vi "N-565 Contol.vi"(0 "N-664 Notifier":refnum<notifier>, 5 "Stage Action":T1={"Action"=enum."Get Position", "Axis"=[], "Setpoint"=[], "Velocity"=0.5, "Cmd Recvd?"=FALSE, "Position"=[], "Status"=enum."Error", "Misc"=variant} {"Velocity" min=0.0 max=1.0 step=0.01}, 11 "VISA In":refnum<visa-resource-name>) -> (4 "N-664 Notifier (Dup)":refnum<notifier>)   [LabVIEW 2016]
uses:
  Stages Controls/Stage Notifier Element.ctl
  Stages Controls/Stage Actions.ctl
  Stages Controls/Stage Status.ctl
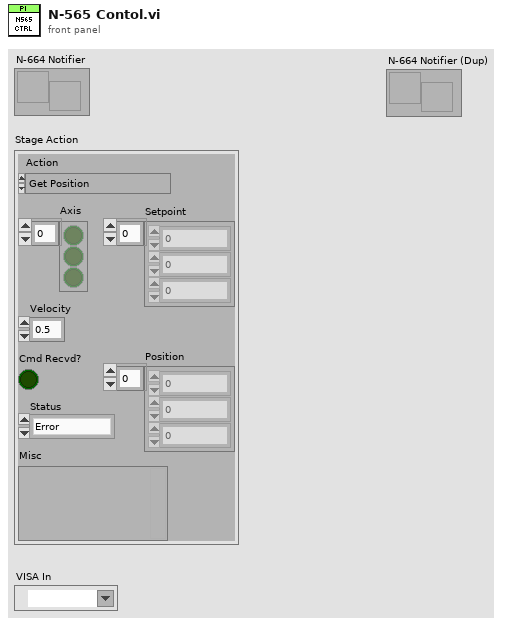
[diagram p1: front panel]
types:
  T1 = typedef "Stage Notifier Element.ctl" = cluster{"Action":T2, "Axis":bool[], "Setpoint":dbl[], "Velocity":dbl, "Cmd Recvd?":bool, "Position":dbl[], "Status":T3, "Misc":variant}
  T2 = typedef "Stage Actions.ctl" = enum16{"Get Position", "MVR", "MOVE", "HALT", "ONTARGET", "ERROR", "REFERENCE", "INIT", "VELOCITY", "STATUS", "EXIT", "HOME", "ZEROPOS", "NANOPOS", "ANALOG", "QUIT"}
  T3 = typedef "Stage Status.ctl" = enum16{"Error", "Abort", "Busy", "On Target"}
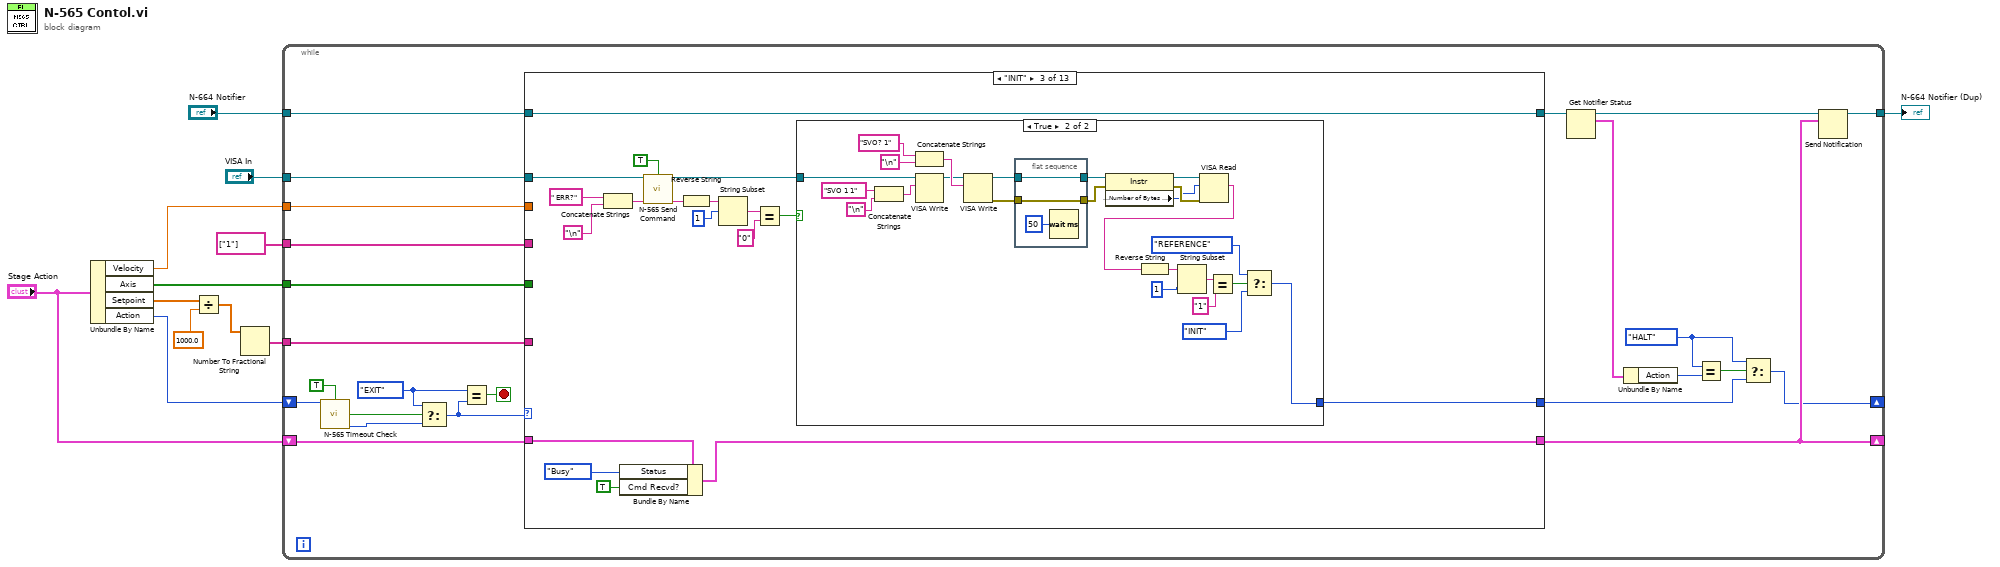
[diagram p0: block diagram]
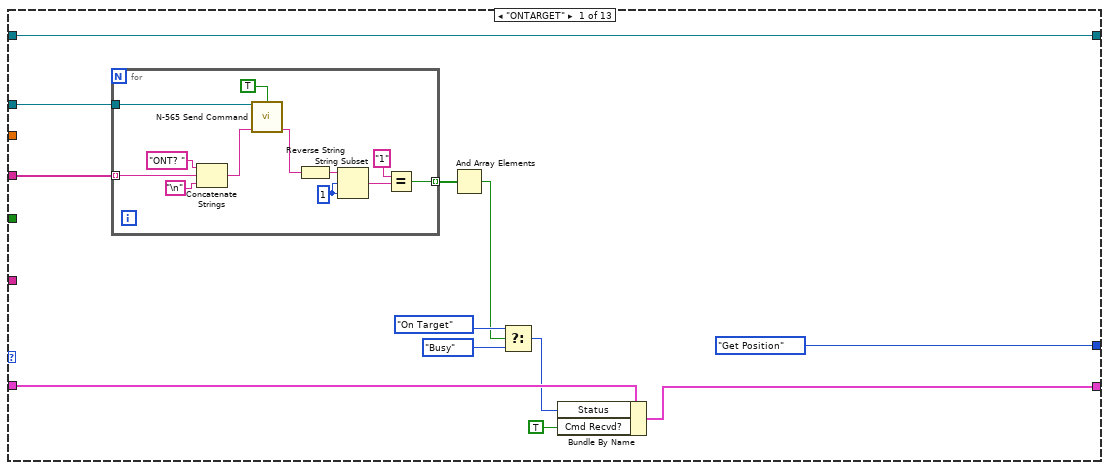
[diagram p2: hidden frame]
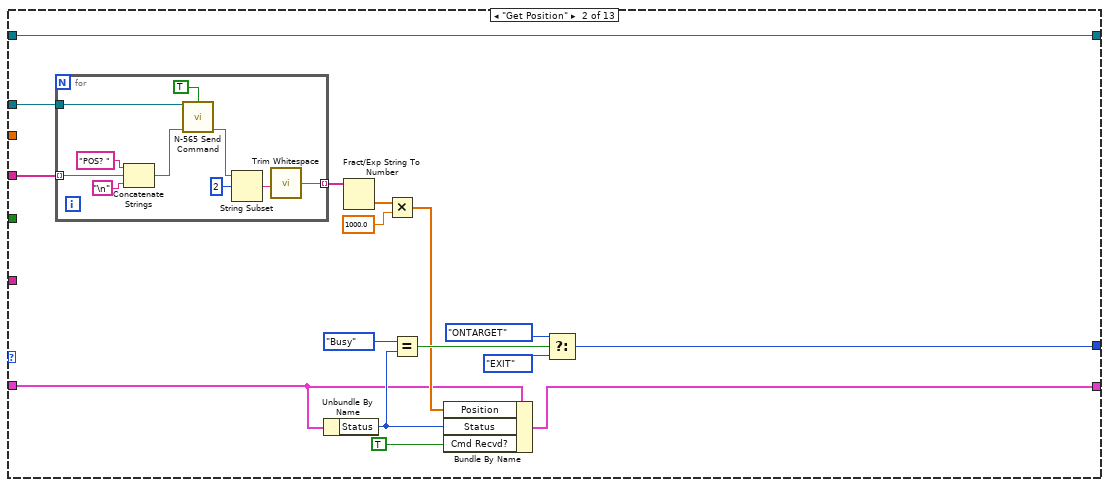
[diagram p3: hidden frame]
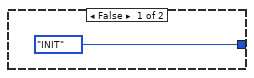
[diagram p4: hidden frame]
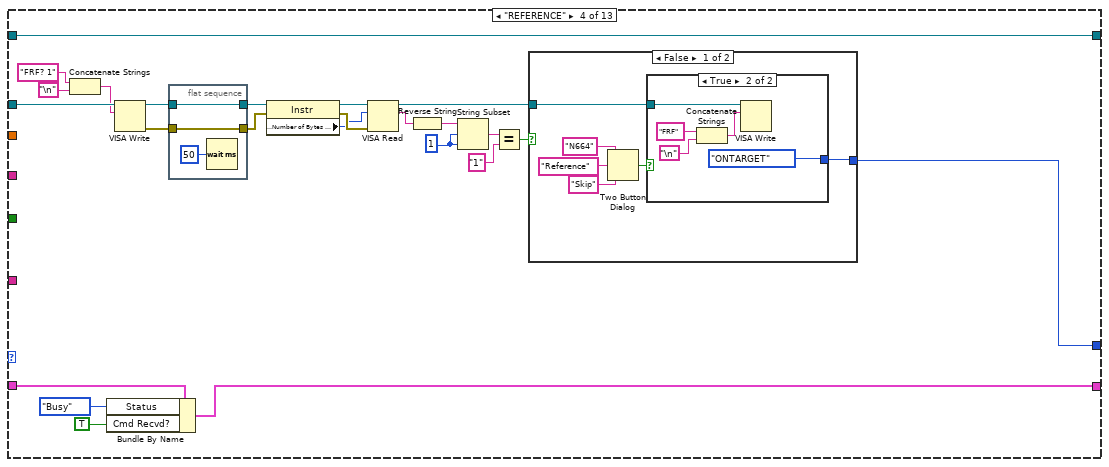
[diagram p5: hidden frame]
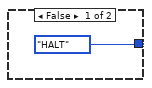
[diagram p6: hidden frame]
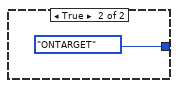
[diagram p7: hidden frame]
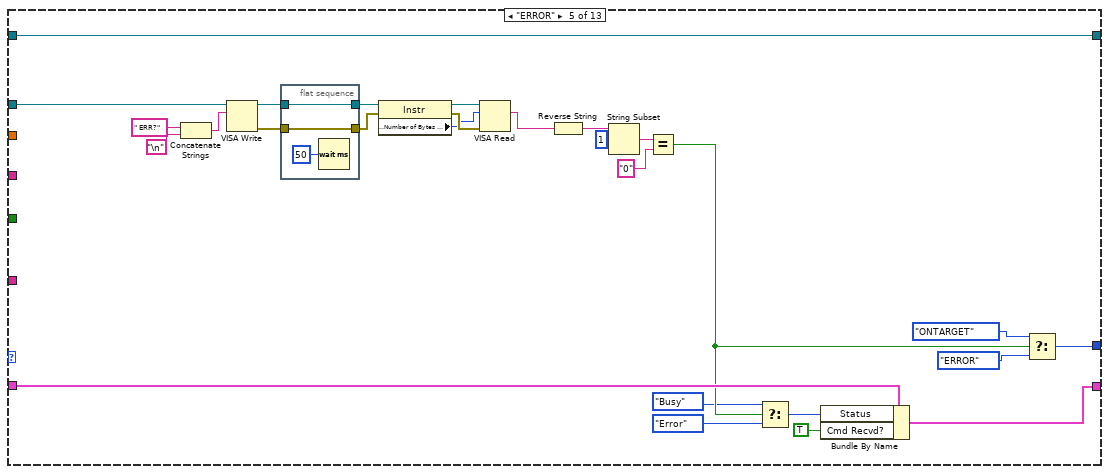
[diagram p8: hidden frame]
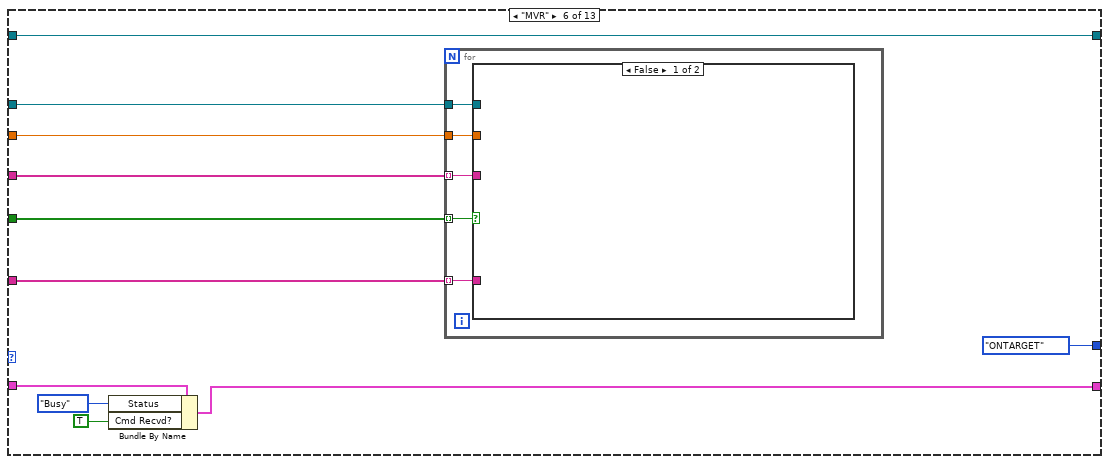
[diagram p9: hidden frame]
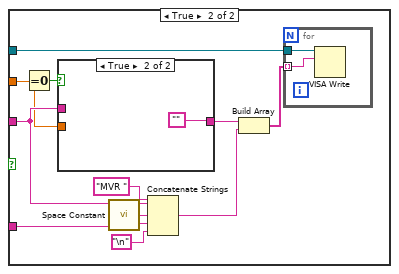
[diagram p10: hidden frame]
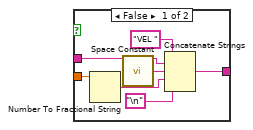
[diagram p11: hidden frame]
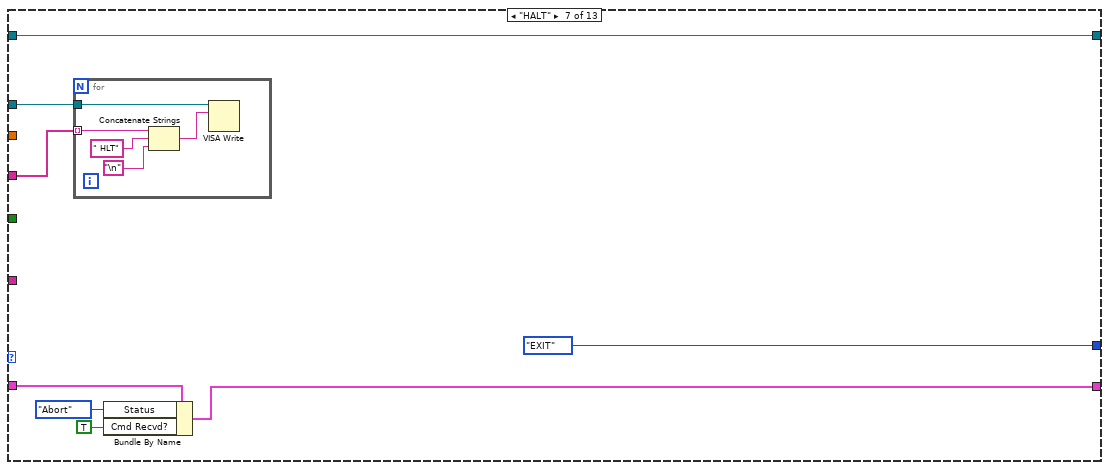
[diagram p12: hidden frame]
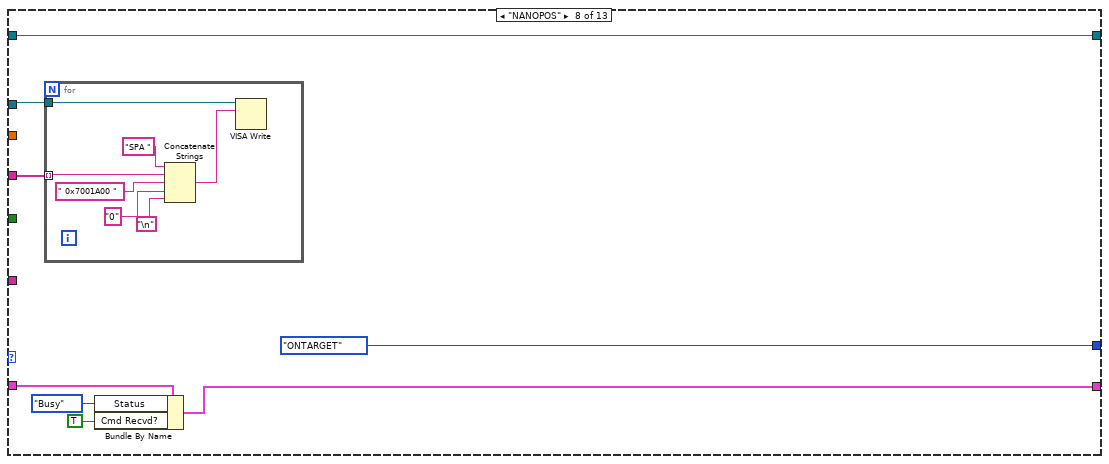
[diagram p13: hidden frame]
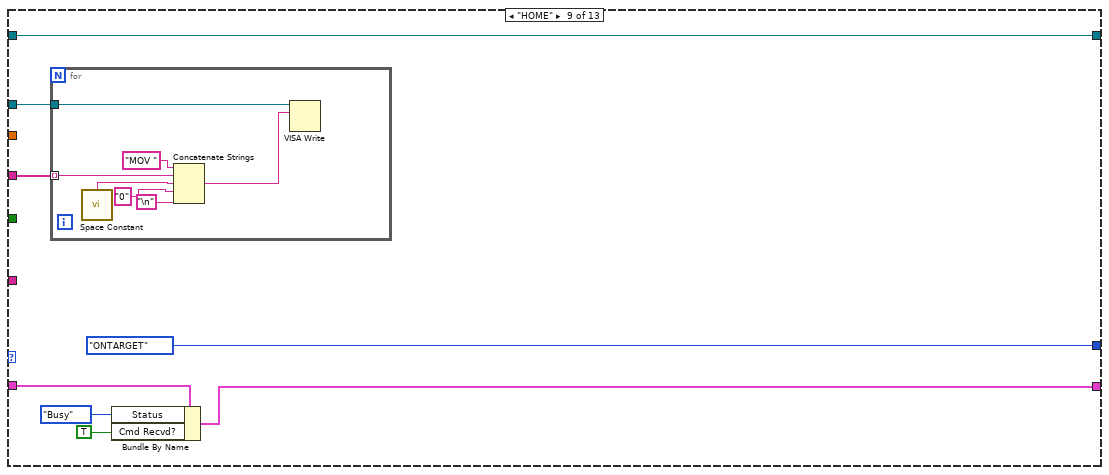
[diagram p14: hidden frame]
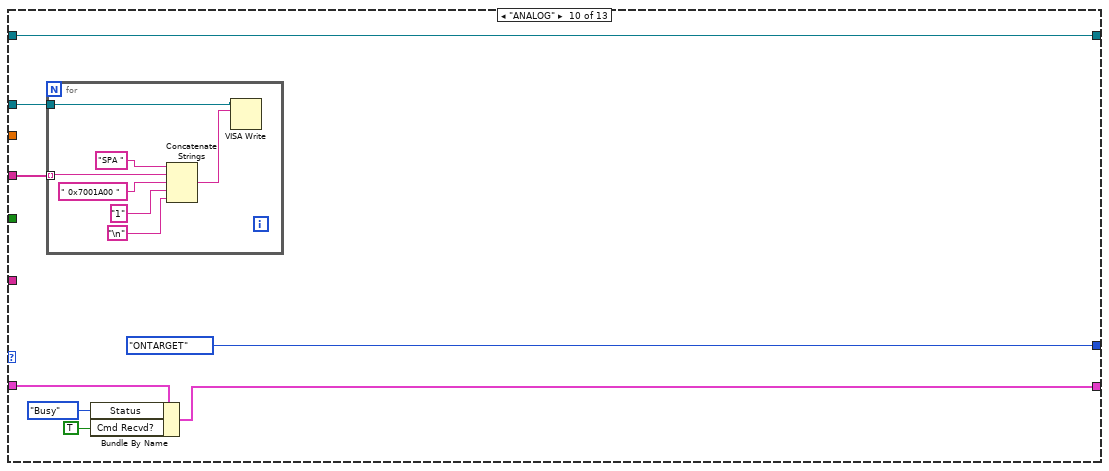
[diagram p15: hidden frame]
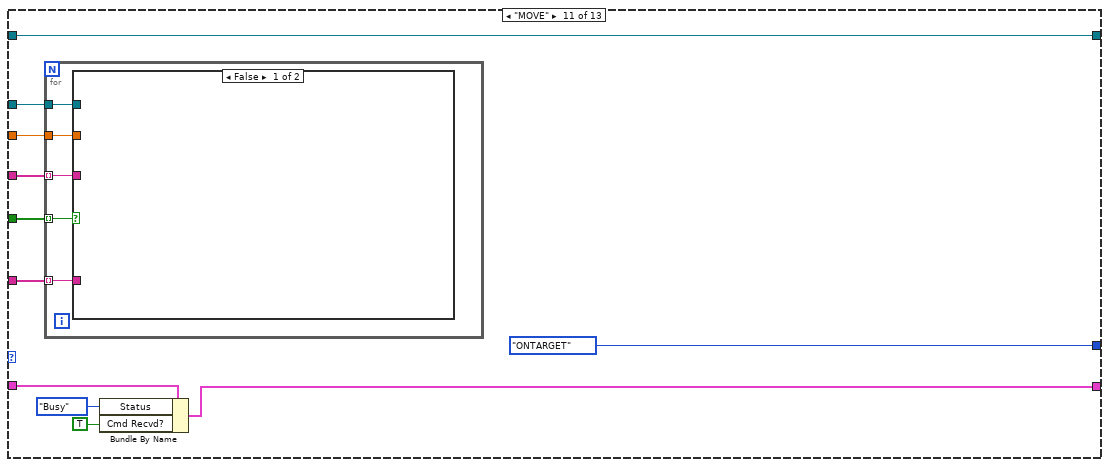
[diagram p16: hidden frame]
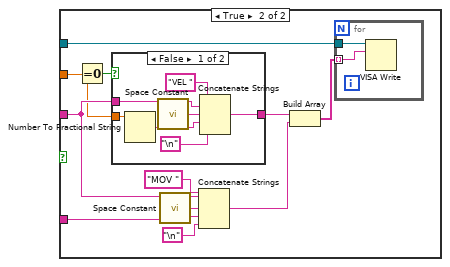
[diagram p17: hidden frame]
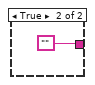
[diagram p18: hidden frame]
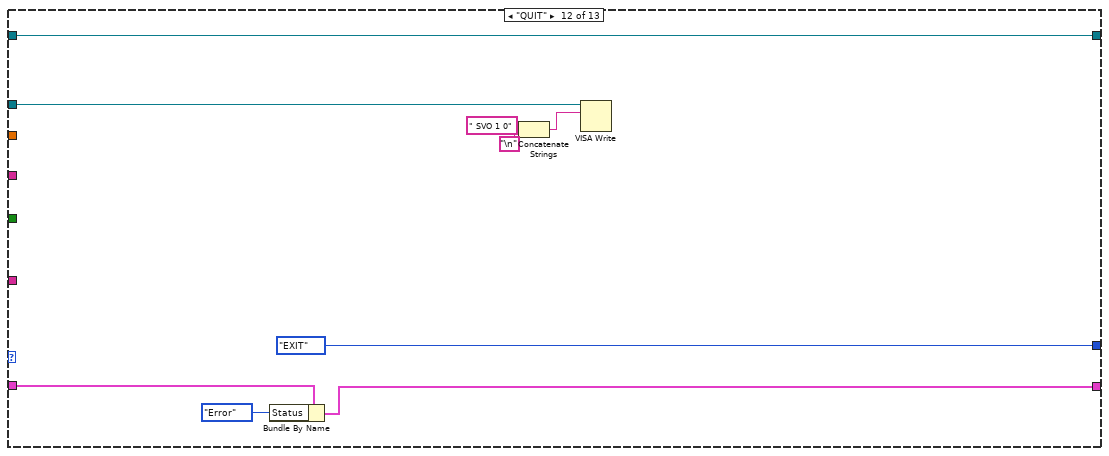
[diagram p19: hidden frame]
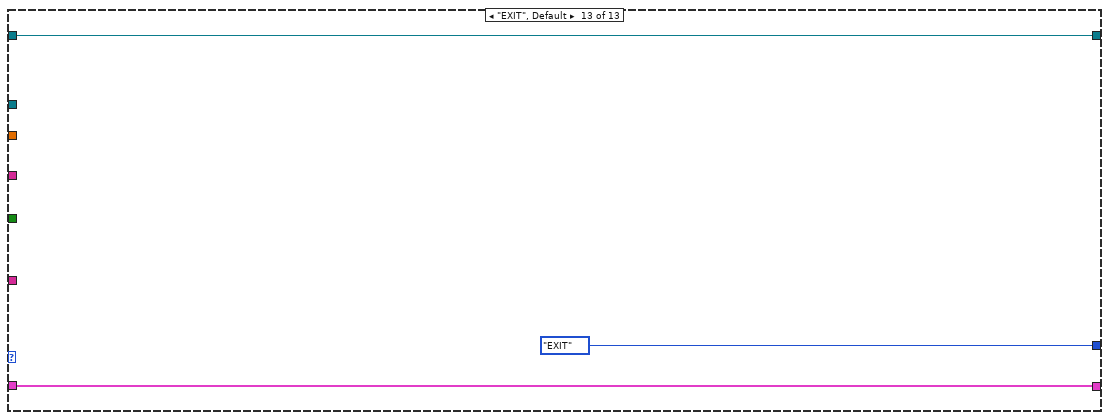
[diagram p20: hidden frame]
diagram:
  n1 = Unbundle By Name("Stage Action") -> ("Velocity"=w10:dbl, "Axis"=w9:bool[], "Setpoint"=w8:dbl[], "Action"=w7:T2)
  n2 = Divide(x=w8, y=1000.0) -> (x/y=w6:dbl[])
  n3 = Number To Fractional String(number=w6) -> (F-format string=w12:string[])  [unwired: 3 in]
  n4 = while {
    tunnel: string[] ["1"] -> [w36]
    shift-right: [w15] -> _
    shift-left: w7 -> [w28]
    tunnel: w9 -> [w34]
    tunnel: w10 -> [w33]
    tunnel: w12 -> [w35]
    shift-right: [w30] -> _
    shift-left: "Stage Action" -> [w32]
    tunnel: "N-664 Notifier" -> [w22]
    tunnel: "VISA In" -> [w14]
    tunnel: [w13] -> w1
    stop <- w23 stop-if-true
    w18 = Stage_Actions."HALT" ("Action")
    w27 = Stage_Actions."EXIT" ("t")
    n5 = call "N-565 Timeout Check.vi"("Action"=w28, "User Input?"=TRUE) -> ("Timeout?"=w26:bool, "Action (Dup)"=w25:T2)  [unwired: 12 in]
    n6 = Select(t=w27, s=w26, f=w25) -> (s? t:f=w24:T2)
    n7 = Equal?(x=w27, y=w24) -> (x = y?=w23:bool)
    n8 = case shown="\"INIT\"" w24 {
      tunnel: w36 -> [w48 w76 _ _ _ w213 w247 w260 w275 w290 w308 _ _]
      tunnel: w14 -> [w37 w63 w92 w151 w177 w205 w241 w254 w269 w284 w298 w336 _]
      tunnel: w35 -> [_ _ _ _ _ w212 _ _ _ _ w307 _ _]
      tunnel: w34 -> [_ _ _ _ _ w211 _ _ _ _ w306 _ _]
      tunnel: w33 -> [_ _ _ _ _ w210 _ _ _ _ w305 _ _]
      tunnel: [Stage_Actions."Get Position" ("Action") w74 w104 w152 w193 Stage_Actions."ONTARGET" ("Action") Stage_Actions."EXIT" ("Action") Stage_Actions."ONTARGET" ("Action") Stage_Actions."ONTARGET" ("Action") Stage_Actions."ONTARGET" ("Action") Stage_Actions."ONTARGET" ("Action") Stage_Actions."EXIT" ("Action") Stage_Actions."EXIT" ("Action")] -> w31
      tunnel: w32 -> [w42 w61 w93 w154 w188 w207 w244 w257 w272 w287 w302 w342 w345]
      tunnel: [w38 w72 w101 w153 w190 w203 w243 w256 w271 w286 w301 w341 w345] -> w30
      tunnel: w22 -> [w39 w62 w87 w133 w173 w204 w240 w253 w268 w283 w299 w335 w344]
      tunnel: [w39 w62 w87 w133 w173 w204 w240 w253 w268 w283 w299 w335 w344] -> w17
      frame "ONTARGET" {
        n9 = for {
          tunnel: w48 -> [w60] mode=indexing
          tunnel: [w57] -> w47 mode=indexing
          tunnel: w37 -> [w52]
          w53 = 1 ("length (rest)")
          n10 = Concatenate Strings("ONT? " ("string"), w60, "\n") -> (w51:string)
          n11 = call "N-565 Send Command.vi"("VISA Ref"=w52, "Wait for Reply?"=TRUE, "Command"=w51) -> ("Response"=w50:string)  [unwired: 10 in, 2 out]
          n12 = Reverse String(1:w50) -> (0:w54:string)
          n13 = String Subset(string=w54, offset (0)=w53, length (rest)=w53) -> (substring=w59:string)
          n14 = Equal?(x="1", y=w59) -> (x = y?=w57:bool)
        }
        n15 = And Array Elements(Boolean array=w47) -> (logical AND=w43:bool)
        n16 = Select(t=Stage_Status."On Target" ("Status"), s=w43, f=Stage_Status."Busy" ("Status")) -> (s? t:f=w41:T3)
        n17 = Bundle By Name(cluster=w42, "Status"=w41, "Cmd Recvd?"=TRUE) -> (w38:T1)
      }
      frame "Get Position" {
        n18 = for {
          tunnel: w76 -> [w86] mode=indexing
          tunnel: [w85] -> w75 mode=indexing
          tunnel: w63 -> [w80]
          n19 = Concatenate Strings("POS? " ("string"), w86, "\n") -> (w78:string)
          n20 = call "N-565 Send Command.vi"("VISA Ref"=w80, "Wait for Reply?"=TRUE, "Command"=w78) -> ("Response"=w79:string)  [unwired: 10 in, 2 out]
          n21 = String Subset(string=w79, offset (0)=2) -> (substring=w81:string)  [unwired: 1 in]
          n22 = call <vilib>:"Trim Whitespace.vi"("string"=w81) -> ("trimmed string"=w85:string)  [unwired: 1 in]
        }
        n23 = Unbundle By Name(w61) -> ("Status"=w69:T3)
        n24 = Fract/Exp String To Number(string=w75) -> (number=w71:dbl[])  [unwired: 3 in, 1 out]
        n25 = Multiply(x=w71, y=1000.0) -> (x*y=w65:dbl[])
        n26 = Equal?(x=Stage_Status."Busy", y=w69) -> (x = y?=w68:bool)
        n27 = Bundle By Name(cluster=w61, "Position"=w65, "Status"=w69, "Cmd Recvd?"=TRUE) -> (w72:T1)
        n28 = Select(t=Stage_Actions."ONTARGET" ("Action"), s=w68, f=Stage_Actions."EXIT" ("Action")) -> (s? t:f=w74:T2)
      }
      frame "INIT" {
        n29 = Concatenate Strings(" ERR?" ("string"), "\n") -> (w89:string)
        n30 = Bundle By Name(cluster=w93, "Status"=Stage_Status."Busy", "Cmd Recvd?"=TRUE) -> (w101:T1)
        n31 = call "N-565 Send Command.vi"("VISA Ref"=w92, "Wait for Reply?"=TRUE, "Command"=w89) -> ("VISA Ref Out"=w91:refnum<visa-resource-name>, "Response"=w90:string)  [unwired: 10 in, 1 out]
        n32 = Reverse String(1:w90) -> (0:w97:string)
        n33 = String Subset(string=w97, offset (0)=1) -> (substring=w95:string)  [unwired: 1 in]
        n34 = Equal?(x=w95, y="0") -> (x = y?=w94:bool)
        n35 = case shown="True" w94 {
          tunnel: [Stage_Actions."INIT" ("Action") w106] -> w104
          tunnel: w91 -> [_ w121]
          frame False {
          }
          frame True {
            w126 = 1 ("length (rest)")
            n36 = Concatenate Strings("SVO 1 1" ("string"), "\n") -> (w128:string)
            n37 = Concatenate Strings("SVO? 1" ("string"), "\n") -> (w112:string)
            n38 = VISA Write(VISA resource name=w121, write buffer=w128) -> (VISA resource name out=w111:refnum<visa-resource-name>)  [unwired: 1 in, 2 out]
            n39 = VISA Write(VISA resource name=w111, write buffer=w112) -> (VISA resource name out=w119:refnum<visa-resource-name>, error out=w118:errorcluster)  [unwired: 1 in, 1 out]
            n40 = flat-sequence {
              tunnel: w119 -> [w131]
              tunnel: w118 -> [w130]
              tunnel: [w131] -> w117
              tunnel: [w130] -> w116
              frame #0 {
                n41 = Wait (ms)(milliseconds to wait=u32 50) -> ()  [unwired: 1 out]
              }
            }
            n42 = property class="Instr"(reference=w117, error in=w116) -> (reference out=w115:refnum<visa-resource-name>, error out=w114:errorcluster, "Serial Settings:Number of Bytes at Serial Port"=w113:u32)
            n43 = VISA Read(VISA resource name=w115, byte count=w113, error in (no error)=w114) -> (read buffer=w110:string)  [unwired: 3 out]
            n44 = Reverse String(1:w110) -> (0:w125:string)
            n45 = String Subset(string=w125, offset (0)=w126, length (rest)=w126) -> (substring=w123:string)
            n46 = Equal?(x=w123, y="1") -> (x = y?=w109:bool)
            n47 = Select(t=Stage_Actions."REFERENCE" ("Action"), s=w109, f=Stage_Actions."INIT" ("Action")) -> (s? t:f=w106:T2)
          }
        }
      }
      frame "REFERENCE" {
        w137 = 1 ("length (rest)")
        n48 = Concatenate Strings("FRF? 1" ("string"), "\n") -> (w141:string)
        n49 = Bundle By Name(cluster=w154, "Status"=Stage_Status."Busy", "Cmd Recvd?"=TRUE) -> (w153:T1)
        n50 = VISA Write(VISA resource name=w151, write buffer=w141) -> (VISA resource name out=w150:refnum<visa-resource-name>, error out=w149:errorcluster)  [unwired: 1 in, 1 out]
        n51 = flat-sequence {
          tunnel: w150 -> [w171]
          tunnel: w149 -> [w170]
          tunnel: [w171] -> w148
          tunnel: [w170] -> w147
          frame #0 {
            n52 = Wait (ms)(milliseconds to wait=u32 50) -> ()  [unwired: 1 out]
          }
        }
        n53 = property class="Instr"(reference=w148, error in=w147) -> (reference out=w146:refnum<visa-resource-name>, error out=w145:errorcluster, "Serial Settings:Number of Bytes at Serial Port"=w144:u32)
        n54 = VISA Read(VISA resource name=w146, byte count=w144, error in (no error)=w145) -> (VISA resource name out=w135:refnum<visa-resource-name>, read buffer=w136:string)  [unwired: 2 out]
        n55 = Reverse String(1:w136) -> (0:w138:string)
        n56 = String Subset(string=w138, offset (0)=w137, length (rest)=w137) -> (substring=w140:string)
        n57 = Equal?(x=w140, y="1") -> (x = y?=w134:bool)
        n58 = case shown="False" w134 {
          tunnel: [w158 Stage_Actions."ONTARGET" ("t")] -> w152
          tunnel: w135 -> [w157 _]
          frame False {
            n59 = Two Button Dialog(message="N664", 1:"Skip" ("F button name (\"Cancel\")"), 2:"Reference" ("T button name (\"OK\")")) -> (T button?=w159:bool)
            n60 = case shown="True" w159 {
              tunnel: [Stage_Actions."HALT" ("Action") Stage_Actions."ONTARGET" ("Action")] -> w158
              tunnel: w157 -> [_ w164]
              frame False {
              }
              frame True {
                n61 = Concatenate Strings("FRF" ("string"), "\n") -> (w166:string)
                n62 = VISA Write(VISA resource name=w164, write buffer=w166) -> ()  [unwired: 1 in, 3 out]
              }
            }
          }
          frame True {
          }
        }
      }
      frame "ERROR" {
        n63 = Concatenate Strings(" ERR?" ("string"), "\n") -> (w176:string)
        n64 = VISA Write(VISA resource name=w177, write buffer=w176) -> (VISA resource name out=w184:refnum<visa-resource-name>, error out=w183:errorcluster)  [unwired: 1 in, 1 out]
        n65 = flat-sequence {
          tunnel: w184 -> [w201]
          tunnel: w183 -> [w200]
          tunnel: [w201] -> w182
          tunnel: [w200] -> w181
          frame #0 {
            n66 = Wait (ms)(milliseconds to wait=u32 50) -> ()  [unwired: 1 out]
          }
        }
        n67 = property class="Instr"(reference=w182, error in=w181) -> (reference out=w180:refnum<visa-resource-name>, error out=w179:errorcluster, "Serial Settings:Number of Bytes at Serial Port"=w178:u32)
        n68 = VISA Read(VISA resource name=w180, byte count=w178, error in (no error)=w179) -> (read buffer=w175:string)  [unwired: 3 out]
        n69 = Reverse String(1:w175) -> (0:w196:string)
        n70 = String Subset(string=w196, offset (0)=1) -> (substring=w194:string)  [unwired: 1 in]
        n71 = Equal?(x=w194, y="0") -> (x = y?=w187:bool)
        n72 = Select(t=Stage_Status."Busy" ("Status"), s=w187, f=Stage_Status."Error" ("Status")) -> (s? t:f=w186:T3)
        n73 = Bundle By Name(cluster=w188, "Status"=w186, "Cmd Recvd?"=TRUE) -> (w190:T1)
        n74 = Select(t=Stage_Actions."ONTARGET" ("Action"), s=w187, f=Stage_Actions."ERROR") -> (s? t:f=w193:T2)
      }
      frame "MVR" {
        n75 = Bundle By Name(cluster=w207, "Status"=Stage_Status."Busy", "Cmd Recvd?"=TRUE) -> (w203:T1)
        n76 = for {
          tunnel: w213 -> [w218] mode=indexing
          tunnel: w212 -> [w217] mode=indexing
          tunnel: w211 -> [w216] mode=indexing
          tunnel: w210 -> [w215]
          tunnel: w205 -> [w214]
          n77 = case shown="False" w216 {
            tunnel: w218 -> [_ w225]
            tunnel: w217 -> [_ w226]
            tunnel: w214 -> [_ w219]
            tunnel: w215 -> [_ w224]
            frame False {
            }
            frame True {
              n78 = Equal To 0?(x=w224) -> (x = 0?=w223:bool)
              n79 = case shown="True" w223 {
                tunnel: w225 -> [w235 _]
                tunnel: w224 -> [w232 _]
                tunnel: [w234 ""] -> w222
                frame False {
                  n80 = Number To Fractional String(number=w232) -> (F-format string=w233:string)  [unwired: 3 in]
                  n81 = call <vilib>:"Space Constant.vi"() -> ("String"=w238:string)
                  n82 = Concatenate Strings("VEL ", w235, w238, w233, "\n") -> (w234:string)
                }
                frame True {
                }
              }
              n83 = call <vilib>:"Space Constant.vi"() -> ("String"=w227:string)
              n84 = Concatenate Strings("MVR ", w225, w227, w226, "\n") -> (w221:string)
              n85 = Build Array(w222, w221) -> (w220:string[])
              n86 = for {
                tunnel: w220 -> [w231] mode=indexing
                tunnel: w219 -> [w230]
                n87 = VISA Write(VISA resource name=w230, write buffer=w231) -> ()  [unwired: 1 in, 3 out]
              }
            }
          }
        }
      }
      frame "HALT" {
        n88 = for {
          tunnel: w247 -> [w249] mode=indexing
          tunnel: w241 -> [w248]
          n89 = Concatenate Strings(w249, " HLT" ("string"), "\n") -> (w250:string)
          n90 = VISA Write(VISA resource name=w248, write buffer=w250) -> ()  [unwired: 1 in, 3 out]
        }
        n91 = Bundle By Name(cluster=w244, "Status"=Stage_Status."Abort", "Cmd Recvd?"=TRUE) -> (w243:T1)
      }
      frame "NANOPOS" {
        n92 = for {
          tunnel: w260 -> [w264] mode=indexing
          tunnel: w254 -> [w261]
          n93 = Concatenate Strings("SPA " ("string"), w264, " 0x7001A00 " ("string"), "0", "\n") -> (w262:string)
          n94 = VISA Write(VISA resource name=w261, write buffer=w262) -> ()  [unwired: 1 in, 3 out]
        }
        n95 = Bundle By Name(cluster=w257, "Status"=Stage_Status."Busy", "Cmd Recvd?"=TRUE) -> (w256:T1)
      }
      frame "HOME" {
        n96 = for {
          tunnel: w275 -> [w278] mode=indexing
          tunnel: w269 -> [w276]
          n97 = call <vilib>:"Space Constant.vi"() -> ("String"=w279:string)
          n98 = Concatenate Strings("MOV " ("string"), w278, w279, "0" ("string"), "\n") -> (w277:string)
          n99 = VISA Write(VISA resource name=w276, write buffer=w277) -> ()  [unwired: 1 in, 3 out]
        }
        n100 = Bundle By Name(cluster=w272, "Status"=Stage_Status."Busy", "Cmd Recvd?"=TRUE) -> (w271:T1)
      }
      frame "ANALOG" {
        n101 = for {
          tunnel: w290 -> [w294] mode=indexing
          tunnel: w284 -> [w291]
          n102 = Concatenate Strings("SPA " ("string"), w294, " 0x7001A00 " ("string"), "1", "\n") -> (w293:string)
          n103 = VISA Write(VISA resource name=w291, write buffer=w293) -> ()  [unwired: 1 in, 3 out]
        }
        n104 = Bundle By Name(cluster=w287, "Status"=Stage_Status."Busy", "Cmd Recvd?"=TRUE) -> (w286:T1)
      }
      frame "MOVE" {
        n105 = for {
          tunnel: w308 -> [w313] mode=indexing
          tunnel: w307 -> [w312] mode=indexing
          tunnel: w306 -> [w311] mode=indexing
          tunnel: w305 -> [w310]
          tunnel: w298 -> [w309]
          n106 = case shown="False" w311 {
            tunnel: w313 -> [_ w320]
            tunnel: w312 -> [_ w321]
            tunnel: w309 -> [_ w314]
            tunnel: w310 -> [_ w319]
            frame False {
            }
            frame True {
              n107 = Equal To 0?(x=w319) -> (x = 0?=w318:bool)
              n108 = case shown="False" w318 {
                tunnel: w320 -> [w330 _]
                tunnel: w319 -> [w327 _]
                tunnel: [w329 ""] -> w317
                frame False {
                  n109 = Number To Fractional String(number=w327) -> (F-format string=w328:string)  [unwired: 3 in]
                  n110 = call <vilib>:"Space Constant.vi"() -> ("String"=w333:string)
                  n111 = Concatenate Strings("VEL ", w330, w333, w328, "\n") -> (w329:string)
                }
                frame True {
                }
              }
              n112 = call <vilib>:"Space Constant.vi"() -> ("String"=w322:string)
              n113 = Concatenate Strings("MOV ", w320, w322, w321, "\n") -> (w316:string)
              n114 = Build Array(w317, w316) -> (w315:string[])
              n115 = for {
                tunnel: w315 -> [w326] mode=indexing
                tunnel: w314 -> [w325]
                n116 = VISA Write(VISA resource name=w325, write buffer=w326) -> ()  [unwired: 1 in, 3 out]
              }
            }
          }
        }
        n117 = Bundle By Name(cluster=w302, "Status"=Stage_Status."Busy", "Cmd Recvd?"=TRUE) -> (w301:T1)
      }
      frame "QUIT" {
        n118 = Bundle By Name(cluster=w342, "Status"=Stage_Status."Error") -> (w341:T1)
        n119 = Concatenate Strings(" SVO 1 0" ("string"), "\n") -> (w339:string)
        n120 = VISA Write(VISA resource name=w336, write buffer=w339) -> ()  [unwired: 1 in, 3 out]
      }
      frame "EXIT", Default {
      }
    }
    n121 = Get Notifier Status(notifier=w17) -> (notifier out=w21:refnum<notifier>, current notification=w16:T1)  [unwired: 1 in, 3 out]
    n122 = Unbundle By Name(w16) -> ("Action"=w19:T2)
    n123 = Equal?(x=w18, y=w19) -> (x = y?=w20:bool)
    n124 = Select(t=w18, s=w20, f=w31) -> (s? t:f=w15:T2)
    n125 = Send Notification(notification=w30, notifier=w21) -> (notifier out=w13:refnum<notifier>)  [unwired: 1 in, 1 out]
  }
  "N-664 Notifier (Dup)" <- w1
